vi "AnnotationList.vi"(9 "y array":dbl[](array[numeric]), 10 "x array":dbl[](array[numeric]), 11 "annotations":dbl[](array[numeric])) -> (3 "annotation list":T1(array[cluster]))   [LabVIEW 2011]
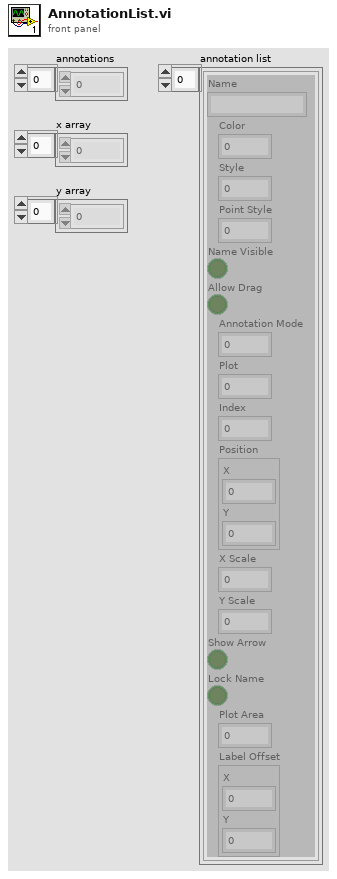
[diagram p1: front panel]
types:
  T1 = cluster{"Name":string, "Color":u32, "Style":u8, "Point Style":u8, "Name Visible":bool, "Allow Drag":bool, "Annotation Mode":u32, "Plot":i32, "Index":i32, "Position":cluster{"X":dbl, "Y":dbl}, "X Scale":u32, "Y Scale":u32, "Show Arrow":bool, "Lock Name":bool, "Plot Area":i32, "Label Offset":cluster{"X":dbl, "Y":dbl}}[]
  T2 = cluster{"Name":string, "Color":u32, "Style":u8, "Point Style":u8, "Name Visible":bool, "Allow Drag":bool, "Annotation Mode":u32, "Plot":i32, "Index":i32, "Position":cluster{"X":dbl, "Y":dbl}, "X Scale":u32, "Y Scale":u32, "Show Arrow":bool, "Lock Name":bool, "Plot Area":i32, "Label Offset":cluster{"X":dbl, "Y":dbl}}
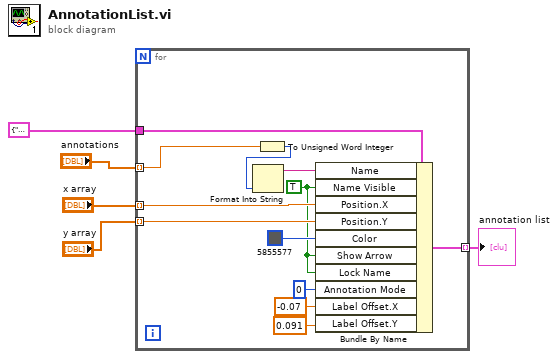
[diagram p0: block diagram]
diagram:
  n1 = for {
    tunnel: "y array" -> [w16] mode=indexing
    tunnel: "x array" -> [w15] mode=indexing
    tunnel: T2 {"Name"="", "Color"=16448250, "Style"=0, "Point Style"=0, "Name Visible"=FALSE, "Allow Drag"=FALSE, "Annotation Mode"=1, "Plot"=0, "Index"=0, "Position"={"X"=0.0, "Y"=0.0}, "X Scale"=0, "Y Scale"=0, "Show Arrow"=FALSE, "Lock Name"=FALSE, "Plot Area"=0, "Label Offset"={"X"=0.0, "Y"=0.0}} ("output cluster") -> [w14]
    tunnel: "annotations" -> [w11] mode=indexing
    tunnel: [w6] -> w5 mode=indexing
    w7 = TRUE ("Name Visible")
    n2 = To Unsigned Word Integer(number=w11) -> (unsigned 16bit integer=w10:u16)
    n3 = Format Into String(w10) -> (resulting string=w17:string)  [unwired: 3 in, 1 out]
    n4 = Bundle By Name(cluster=w14, "Name"=w17, "Name Visible"=w7, "Position.X"=w15, "Position.Y"=w16, "Color"=u32 5855577, "Show Arrow"=w7, "Lock Name"=w7, "Annotation Mode"=u32 0, "Label Offset.X"=-0.07, "Label Offset.Y"=0.091) -> (w6:T2)
  }
  "annotation list" <- w5
